vi "audio test.vi"() -> ()   [LabVIEW 2009]
uses:
  <vilib>/Analysis/NI_AALBase.lvlib
panel:
  out "buffer writes":i32
  in  "STOP":bool
  out "Sinc Pattern":dbl[](graph)
  in  "player controls":cluster{"play/pause":bool, "volume":u16} {"volume" scale=0.0..65535.0}
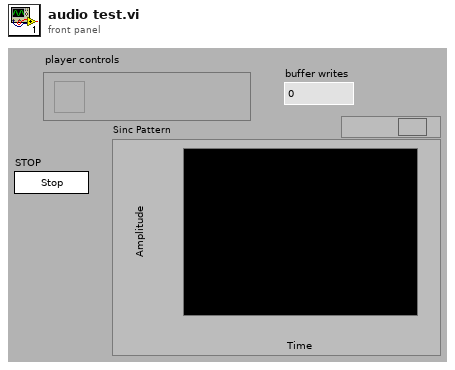
[diagram p1: front panel]
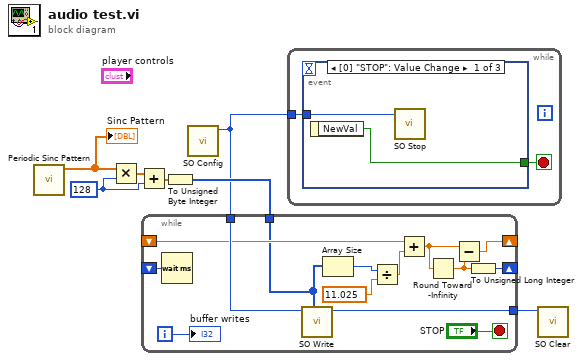
[diagram p0: block diagram]
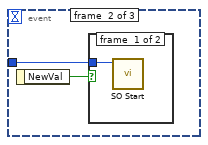
[diagram p2: hidden frame]
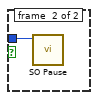
[diagram p3: hidden frame]
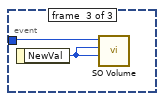
[diagram p4: hidden frame]
diagram:
  w5 = 128
  n1 = call <vilib>:"Periodic Sinc Pattern.vi"() -> ("Periodic Sinc Pattern"=w7:dbl[])  [unwired: 10 in, 1 out]
  "Sinc Pattern" <- w7
  n2 = Multiply(x=w7, y=w5) -> (x*y=w6:dbl[])
  n3 = Add(x=w6, y=w5) -> (x+y=w4:dbl[])
  n4 = To Unsigned Byte Integer(number=w4) -> (unsigned 8bit integer=w3:u8[])
  n5 = call <vilib>:"SO Config.vi"() -> ("task ID out"=w2:u32)  [unwired: 10 in, 1 out]
  n6 = while {
    tunnel: w2 -> [w21]
    tunnel: [w20] -> w1
    shift-right: [w14] -> _
    shift-left: _ -> [w16]
    shift-right: [w12] -> _
    shift-left: _ -> [w11]
    tunnel: w3 -> [w9]
    i -> [w10]
    stop <- "STOP" stop-if-true
    n7 = Wait (ms)(milliseconds to wait=w11) -> ()  [unwired: 1 out]
    n8 = call <vilib>:"SO Write.vi"("mono 8-bit"=w9, "task ID in"=w21) -> ("task ID out"=w20:u32)  [unwired: 8 in, 1 out]
    n9 = Array Size(array=w9) -> (size(s)=w18:i32)
    n10 = Divide(x=w18, y=11.025) -> (x/y=w17:dbl)
    n11 = Add(x=w16, y=w17) -> (x+y=w15:dbl)
    n12 = Round Toward -Infinity(1:w15) -> (0:w13:dbl)
    n13 = Subtract(x=w15, y=w13) -> (x-y=w14:dbl)
    n14 = To Unsigned Long Integer(number=w13) -> (unsigned 32bit integer=w12:u32)
    "buffer writes" <- w10
  }
  n15 = while {
    tunnel: w2 -> [w22]
    stop <- w23 stop-if-true
    n16 = event shown="[0] \"STOP\": Value Change" {
      selector: _ -> [_ _ _]
      dyn-events: _ -> [_ _ _]
      timeout: _ -> [_ _ _]
      tunnel: [w25 _ _] -> w23
      tunnel: w22 -> [w24 w26 w31]
      event #0 {
        n17 = event-data() -> ("NewVal"=w25:bool)  [unwired: 1 in]
        n18 = call <vilib>:"SO Stop.vi"("task ID in"=w24) -> ()  [unwired: 9 in, 2 out]
      }
      event #1 {
        n19 = event-data() -> ("NewVal"=w27:bool)  [unwired: 1 in]
        n20 = case shown="False" w27 {
          tunnel: w26 -> [w28 w29]
          frame #0 {
            n21 = call <vilib>:"SO Start.vi"("task ID in"=w28) -> ()  [unwired: 9 in, 2 out]
          }
          frame #1 {
            n22 = call <vilib>:"SO Pause.vi"("task ID in"=w29) -> ()  [unwired: 9 in, 2 out]
          }
        }
      }
      event #2 {
        n23 = event-data() -> ("NewVal"=w30:u16)  [unwired: 1 in]
        n24 = call <vilib>:"SO Volume.vi"("right channel"=w30, "left channel"=w30, "task ID in"=w31) -> ()  [unwired: 7 in, 2 out]
      }
    }
  }
  n25 = call <vilib>:"SO Clear.vi"("task ID in"=w1) -> ()  [unwired: 10 in, 1 out]
